vi "Register gRPC Methods.vi"(8 "error in (no error)":errorcluster, 11 "Template Server in":refnum<class "QueryServer.lvclass">) -> (0 "error out":errorcluster, 3 "Template Server out":refnum<class "QueryServer.lvclass">)   [LabVIEW 2019, in "Query_server.lvlib" / "QueryServer.lvclass"]
uses:
  QueryServer.lvclass
  QueryServer.lvclass/QueryServer.ctl
  typeDefs/Server Internal UEs.ctl
  typeDefs/Server gRPC UEs.ctl
  <vilib>/gRPC/LabVIEW gRPC Library/Shared/grpcId.ctl
  <vilib>/gRPC/LabVIEW gRPC Library/grpc-lvsupport-release.lvlib
  <vilib>/gRPC/LabVIEW gRPC Library/Server API/typeDefs/gRPCId Cluster.ctl
  typeDefs/Server Internal Message.ctl
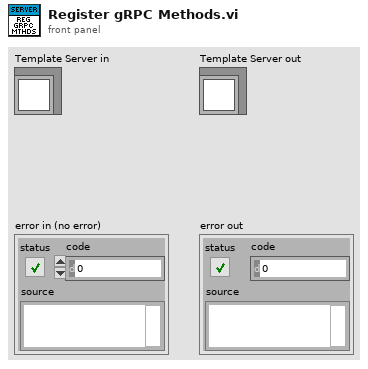
[diagram p1: front panel]
types:
  T1 = typedef "Query_server.lvlib/QueryServer.lvclass/Server gRPC UEs.ctl" = cluster{"queryserver_QueryServer_Invoke gRPC UE":refnum<user-event>, "queryserver_QueryServer_Query gRPC UE":refnum<user-event>, "queryserver_QueryServer_Register gRPC UE":refnum<user-event>}
  T2 = typedef "Query_server.lvlib/QueryServer.lvclass/Server Internal UEs.ctl" = cluster{"queryserver_QueryServer_Invoke Internal UE":refnum<user-event>, "queryserver_QueryServer_Query Internal UE":refnum<user-event>, "queryserver_QueryServer_Register Internal UE":refnum<user-event>}
  T3 = typedef "grpc-lvsupport-release.lvlib/grpcId.ctl" = u64
  T4 = typedef "Query_server.lvlib/QueryServer.lvclass/Server Internal Message UE.ctl" = refnum<user-event>
  T5 = typedef "grpc-lvsupport-release.lvlib/gRPCId Cluster UE.ctl" = refnum<user-event>
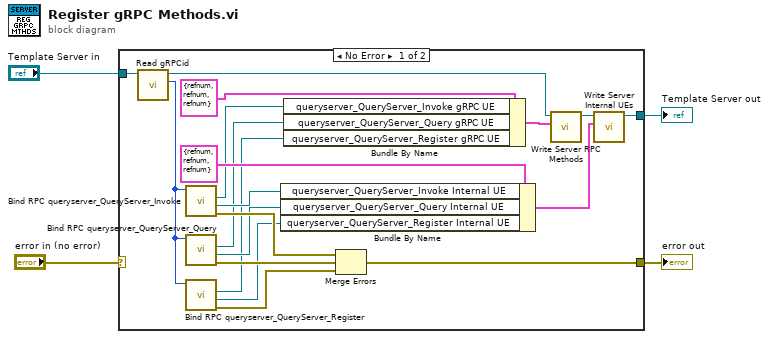
[diagram p0: block diagram]
diagram:
  n1 = case shown="No Error" "error in (no error)" {
    selector: "error in (no error)" -> [_ w24]
    tunnel: "Template Server in" -> [w15 w25]
    tunnel: [w23 w24] -> w3
    tunnel: [w22 w25] -> w2
    frame No Error {
      n2 = call-dynamic "Read gRPCid.vi"("gRPC service in"=w15) -> ("gRPCid"=w14:T3, "gRPC service out"=w16:refnum<class "QueryServer.lvclass">)  [unwired: 8 in, 1 out]
      n3 = call "Bind RPC queryserver_QueryServer_Invoke.vi"("gRPCid server in"=w14) -> ("error out"=w13:errorcluster, "queryserver_QueryServer_Invoke Internal UE"=w12:T4, "queryserver_QueryServer_Invoke gRPC UE"=w11:T5)  [unwired: 7 in, 1 out]
      n4 = call "Bind RPC queryserver_QueryServer_Query.vi"("gRPCid server in"=w14) -> ("error out"=w10:errorcluster, "queryserver_QueryServer_Query Internal UE"=w8:T4, "queryserver_QueryServer_Query gRPC UE"=w9:T5)  [unwired: 7 in, 1 out]
      n5 = call "Bind RPC queryserver_QueryServer_Register.vi"("gRPCid server in"=w14) -> ("error out"=w7:errorcluster, "queryserver_QueryServer_Register Internal UE"=w5:T4, "queryserver_QueryServer_Register gRPC UE"=w6:T5)  [unwired: 7 in, 1 out]
      n6 = Bundle By Name ("Bundle Internal UEs")(cluster=T2 {"queryserver_QueryServer_Invoke Internal UE"=refnum, "queryserver_QueryServer_Query Internal UE"=refnum, "queryserver_QueryServer_Register Internal UE"=refnum} ("Server Internal UEs"), "queryserver_QueryServer_Invoke Internal UE"=w12, "queryserver_QueryServer_Query Internal UE"=w8, "queryserver_QueryServer_Register Internal UE"=w5) -> (w21:T2)
      n7 = Bundle By Name ("Bundle gRPC UEs")(cluster=T1 {"queryserver_QueryServer_Invoke gRPC UE"=refnum, "queryserver_QueryServer_Query gRPC UE"=refnum, "queryserver_QueryServer_Register gRPC UE"=refnum} ("gRPC Server Method Events"), "queryserver_QueryServer_Invoke gRPC UE"=w11, "queryserver_QueryServer_Query gRPC UE"=w9, "queryserver_QueryServer_Register gRPC UE"=w6) -> (w18:T1)
      n8 = Merge Errors(w13, w10, w7) -> (w23:errorcluster)
      n9 = call "Write Server RPC Methods.vi"("Server RPC Methods"=w18, "SignalGeneratorService in"=w16) -> ("SignalGeneratorService out"=w19:refnum<class "QueryServer.lvclass">)  [unwired: 8 in, 1 out]
      n10 = call "Write Server Internal UEs.vi"("Server Internal UEs"=w21, "SignalGeneratorService in"=w19) -> ("SignalGeneratorService out"=w22:refnum<class "QueryServer.lvclass">)  [unwired: 8 in, 1 out]
    }
    frame Error {
    }
  }
  "error out" <- w3
  "Template Server out" <- w2
